vi "Read Suite PublicEvents.vi"(8 "error in (no error)":errorcluster, 11 "Test Suite in":refnum<class "Test Suite.lvclass">) -> (0 "error out":errorcluster, 2 "Test Suite Public Events":T1, 3 "Test Suite out":refnum<class "Test Suite.lvclass">)   [LabVIEW 2013, in "Caraya.lvlib" / "Test Suite.lvclass"]
uses:
  Test Suite.lvclass
  Suite PublicEvents -- cluster.ctl
  Test Result/Test Result.lvclass
  Test Suite.lvclass/Test Suite.ctl
  Test Assert Factory/Test Assert Factory.lvclass/Test Assert Factory.ctl
  Test Assert Factory/Test Assert Factory.lvclass
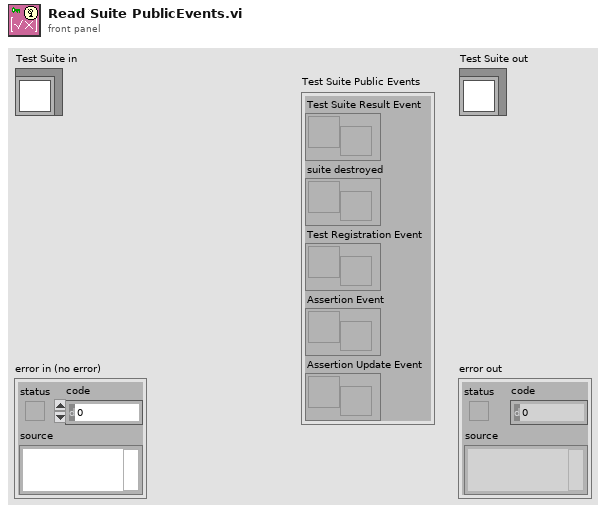
[diagram p1: front panel]
types:
  T1 = typedef "Caraya.lvlib/Test Suite.lvclass/Suite PublicEvents -- cluster.ctl" = cluster{"Test Suite Result Event":refnum<user-event>, "suite destroyed":refnum<user-event>, "Test Registration Event":refnum<user-event>, "Assertion Event":refnum<user-event>, "Assertion Update Event":refnum<user-event>}
  T2 = typedef "Caraya.lvlib/Test Result.lvclass/Test Events -- cluster.ctl" = cluster{"Test Registration Event":refnum<user-event>, "Assertion Event":refnum<user-event>, "Assertion Update Event":refnum<user-event>}
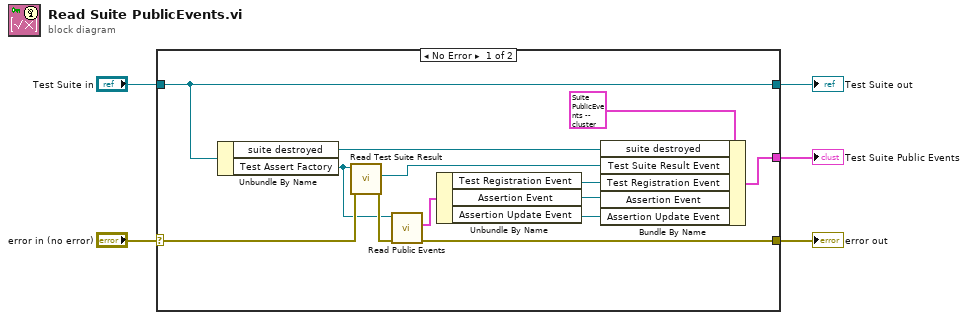
[diagram p0: block diagram]
diagram:
  n1 = case shown="No Error" "error in (no error)" {
    selector: "error in (no error)" -> [w17 w20]
    tunnel: [w7 w20] -> w4
    tunnel: [w18 w19] -> w2
    tunnel: "Test Suite in" -> [w18 w19]
    tunnel: [w13 _] -> w1
    frame No Error {
      n2 = Unbundle By Name(w18) -> ("suite destroyed"=w15:refnum<user-event>, "Test Assert Factory"=w6:refnum<class "Test Assert Factory.lvclass">)
      n3 = call "Read Test Suite Result.vi"("error in (no error)"=w17, "Test Assert Factory in"=w6) -> ("error out"=w8:errorcluster, "Test Suite Result"=w14:refnum<user-event>)  [unwired: 7 in, 1 out]
      n4 = call "Read Public Events.vi"("error in (no error)"=w8, "Test Assert Factory in"=w6) -> ("error out"=w7:errorcluster, "Public Events"=w12:T2)  [unwired: 7 in, 1 out]
      n5 = Unbundle By Name(w12) -> ("Test Registration Event"=w11:refnum<user-event>, "Assertion Event"=w10:refnum<user-event>, "Assertion Update Event"=w9:refnum<user-event>)
      n6 = Bundle By Name(cluster=T1 {"Test Suite Result Event"=refnum, "suite destroyed"=refnum, "Test Registration Event"=refnum, "Assertion Event"=refnum, "Assertion Update Event"=refnum} ("Public Events"), "suite destroyed"=w15, "Test Suite Result Event"=w14, "Test Registration Event"=w11, "Assertion Event"=w10, "Assertion Update Event"=w9) -> (w13:T1)
    }
    frame Error {
    }
  }
  "error out" <- w4
  "Test Suite out" <- w2
  "Test Suite Public Events" <- w1
